vi "KM_HFLI_get_one_data_point.vi"(0 "Handle In":T1 {"Handle" format="0x%08x"; "Conn" format="0x%08x"}, 2 "Freq Sequence In":dbl[](array[numeric]) format="%#_6p", 5 "Error In":errorcluster, 6 "Harmonic (1=fundamental)":i32=1 min=1 max=66000, 7 "Oscillator (0)":u16, 8 "Order (4)":i32(ring)=4 items=["6, 1st"=1, "12, 2nd"=2, "18, 3rd"=3, "24, 4th"=4, "30, 5th"=5, "36, 6th"=6, "42, 7th"=7, "48, 8th"=8], 9 "Input Demods (0)":u16[](array[numeric])=[0], 10 "Averaging":u16(ring)=1 caption="Averaging (1)" items=["1"=1, "2"=2, "4"=4, "8"=8, "16"=16, "32"=32, "64"=64, "128"=128], 11 "Output Demod (0)":u16, 13 "Signal Output (0)":u16 max=1) -> (14 "Handle Out":T1 {"Handle" format="0x%08x"; "Conn" format="0x%08x"}, 17 "Frequency OUT":dbl caption="Frequency (Hz)" format="%_7p", 18 "z OUT":cdb[](array[numeric]), 19 "Error Out":errorcluster)   [LabVIEW 2015]
uses:
  Zurich/Zurich Instruments/LabOne/API/LabVIEW/Zurich Instruments LabOne/Zurich Instruments LabOne.lvlib
  Zurich/Zurich Instruments/LabOne/API/LabVIEW/Zurich Instruments LabOne/Public/Utility/ziTicksToS_single.vi
  Zurich/Zurich Instruments/LabOne/API/LabVIEW/Zurich Instruments LabOne/Public/ziTypeHandle.ctl
panel:
  out "Bandwidth_indic":dbl=100.0 caption="Bandwidth (Hz)" format="%_3p"
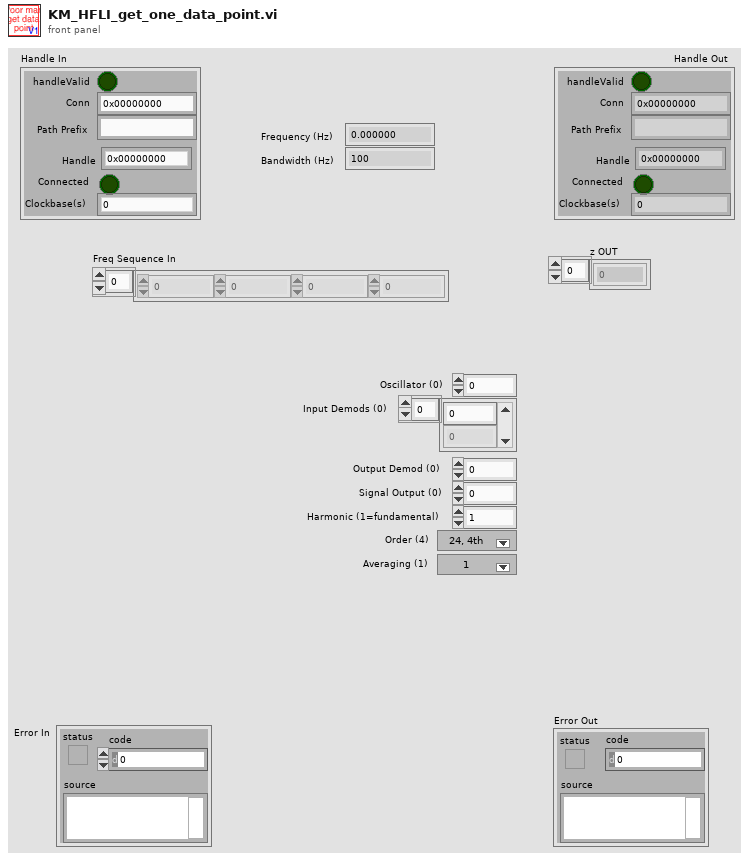
[diagram p1: front panel]
types:
  T1 = typedef "Zurich Instruments LabOne.lvlib/ziTypeHandle.ctl" = cluster{"handleValid":bool, "Conn":u64, "Path Prefix":string, "Handle":u64, "Connected":bool, "Clockbase(s)":dbl}
  T2 = cluster{"Timestamps (ticks)":u64, "X (Vrms)":dbl, "Y (Vrms)":dbl, "Osc Phase (deg)":dbl, "Freq (Hz)":dbl, "DIO":u32, "AuxIn0 (V)":dbl, "AuxIn1 (V)":dbl}
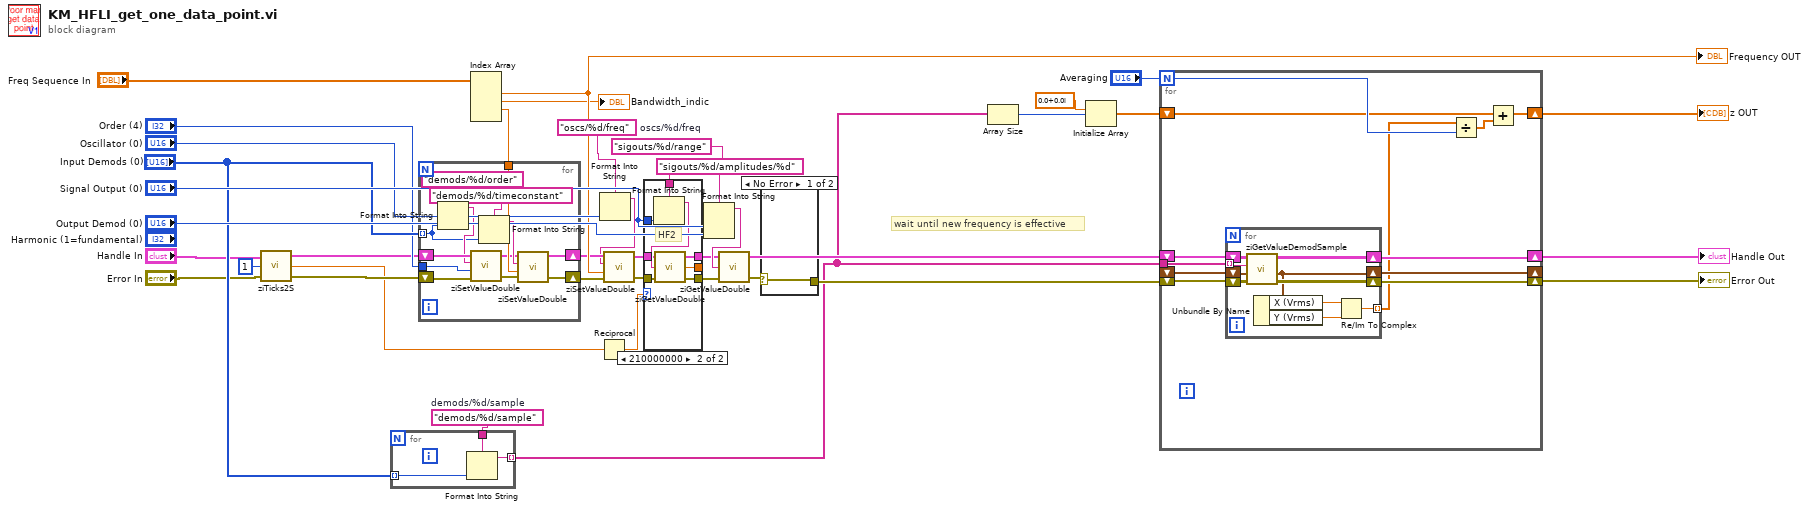
[diagram p0: block diagram]
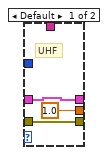
[diagram p2: hidden frame]
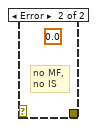
[diagram p3: hidden frame]
diagram:
  w20 = "oscs/%d/freq"  # oscs/%d/freq
  w25 = "demods/%d/sample"  # demods/%d/sample
  # "wait until new frequency is effective"
  n1 = call-poly "ziTicks2S.vi"("Error In"="Error In", "Timestamp(ticks)"=u64 1, "Handle In"="Handle In") -> ("Error Out"=w11:errorcluster, "Timestamp(s)"=w9:dbl, "Handle Out"=w10:T1)
  n2 = for {
    tunnel: w25 -> [w42]
    tunnel: "Input Demods (0)" -> [w41] mode=indexing
    tunnel: [w40] -> w5 mode=indexing
    n3 = Format Into String(format string=w42, w41) -> (resulting string=w40:string)  [unwired: 2 in, 1 out]
  }
  n4 = Index Array(array="Freq Sequence In") -> (element #1=w29:dbl, element #2=→"Bandwidth_indic":dbl, element #3=w21:dbl)  [unwired: 4 in, 1 out]
  "Frequency OUT" <- w29
  n5 = for {
    tunnel: "Input Demods (0)" -> [w43] mode=indexing
    tunnel: w21 -> [w55]
    shift-right: [w52] -> w19
    shift-left: w10 -> [w48]
    shift-right: [w51] -> w18
    shift-left: w11 -> [w49]
    tunnel: "Order (4)" -> [w46]
    n6 = Format Into String(format string="demods/%d/order", w43) -> (resulting string=w44:string)  [unwired: 2 in, 1 out]
    n7 = call "ziSetValueDouble.vi"("Error In"=w49, "Value"=w46, "Path"=w44, "Handle In"=w48) -> ("Error Out"=w50:errorcluster, "Handle Out"=w47:T1)  [unwired: 1 in]
    n8 = Format Into String(format string="demods/%d/timeconstant", w43) -> (resulting string=w53:string)  [unwired: 2 in, 1 out]
    n9 = call "ziSetValueDouble.vi"("Error In"=w50, "Value"=w55, "Path"=w53, "Handle In"=w47) -> ("Error Out"=w51:errorcluster, "Handle Out"=w52:T1)  [unwired: 1 in]
  }
  n10 = Reciprocal(x=w9) -> (1/x=w8:dbl)
  n11 = Format Into String(format string=w20, "Oscillator (0)") -> (resulting string=w17:string)  [unwired: 2 in, 1 out]
  n12 = call "ziSetValueDouble.vi"("Error In"=w18, "Value"=w29, "Path"=w17, "Handle In"=w19) -> ("Error Out"=w14:errorcluster, "Handle Out"=w15:T1)  [unwired: 1 in]
  n13 = case shown="210000000" w8 {
    tunnel: "sigouts/%d/range" -> [_ w65]
    tunnel: "Signal Output (0)" -> [_ w64]
    tunnel: [w56 w63] -> w24
    tunnel: [w58 w62] -> w23
    tunnel: [1.0 ("Value") w61] -> _
    tunnel: w15 -> [w56 w60]
    tunnel: w14 -> [w58 w59]
    frame Default {
      # "UHF"
    }
    frame 210000000 {
      # "HF2"
      n14 = Format Into String(format string=w65, w64) -> (resulting string=w66:string)  [unwired: 2 in, 1 out]
      n15 = call "ziGetValueDouble.vi"("error in"=w59, "Path"=w66, "Handle in"=w60) -> ("error out"=w62:errorcluster, "Value"=w61:dbl, "Handle out"=w63:T1)
    }
  }
  n16 = Format Into String(format string="sigouts/%d/amplitudes/%d", "Signal Output (0)", "Output Demod (0)") -> (resulting string=w27:string)  [unwired: 2 in, 1 out]
  n17 = call "ziGetValueDouble.vi"("error in"=w23, "Path"=w27, "Handle in"=w24) -> ("error out"=w13:errorcluster, "Handle out"=w7:T1)  [unwired: 1 out]
  n18 = case shown="No Error" w13 {
    selector: w13 -> [w67 _]
    tunnel: [w67 _] -> w6
    frame No Error {
    }
    frame Error {
      (unwired) 0.0
      # "no MF,\nno IS"
    }
  }
  n19 = Array Size(array=w5) -> (size(s)=w4:i32)
  n20 = Initialize Array(cdb 0.0+0.0i ("element"), w4) -> (w2:cdb[])
  n21 = for {
    N: "Averaging" -> [w74]
    shift-right: [w79] -> w37
    shift-left: w7 -> [w73]
    shift-right: [w78] -> w36
    shift-left: w6 -> [w71]
    tunnel: w5 -> [w77]
    shift-right: [w76] -> _
    shift-left: _ -> [w72]
    shift-right: [w68] -> w1
    shift-left: w2 -> [w69]
    n22 = for {
      shift-right: [w87] -> w78
      shift-left: w71 -> [w88]
      shift-right: [w86] -> w79
      shift-left: w73 -> [w89]
      shift-right: [w84] -> w76
      shift-left: w72 -> [w85]
      tunnel: w77 -> [w83] mode=indexing
      tunnel: [w80] -> w70 mode=indexing
      n23 = call "ziGetValueDemodSample.vi"("error in"=w88, "Demod Sample In"=w85, "Path"=w83, "Handle In"=w89) -> ("error out"=w87:errorcluster, "Demod Sample Out"=w84:T2, "Handle Out"=w86:T1)  [unwired: 1 in]
      n24 = Unbundle By Name(w84) -> ("X (Vrms)"=w82:dbl, "Y (Vrms)"=w81:dbl)
      n25 = Re/Im To Complex(1:w81, 2:w82) -> (0:w80:cdb)
    }
    n26 = Divide(x=w70, y=w74) -> (x/y=w75:cdb[])
    n27 = Add(x=w69, y=w75) -> (x+y=w68:cdb[])
  }
  "Handle Out" <- w37
  "Error Out" <- w36
  "z OUT" <- w1
